vi "Add Modules.vi"(8 "error in (no error)":errorcluster, 10 "Modules in":refnum<k24>[](array[refnum]), 11 "Item Ref in":T1 format="%.0x") -> (0 "error out":errorcluster, 2 "Modules out":refnum<k24>[](array[refnum]), 3 "Item Ref out":T1 format="%.0x")   [LabVIEW 2014, in "SLSC configuration System Explorer.lvlib"]
uses:
  SLSC configuration System Explorer.lvlib
  C:/Files/Custom VeriStand Development/DET-SPI-Tool/XML Deserializer/SLSC Deserializer/SLSC Deserializer/bin/Release/SLSC Deserializer.dll
  XML Deserializer/SLSC Deserializer/SLSC Deserializer/bin/Release/SLSC Deserializer.dll
  <vilib>/NI Veristand/Custom Device API/Custom Device Item Ref.ctl
  Type Defs/Card Position.ctl
  Shared/SPI Utility/Slot #.ctl
  Shared/SLSC configuration Shared.lvlib
  <vilib>/NI Veristand/Custom Device API/Custom Device API.lvlib
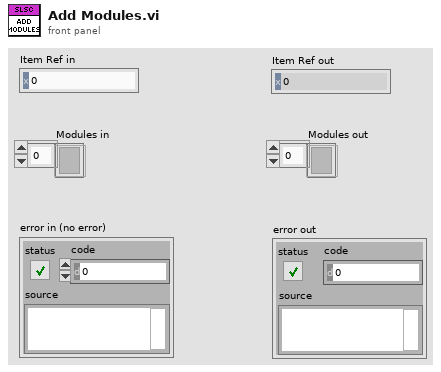
[diagram p1: front panel]
types:
  T1 = typedef "Custom Device API.lvlib/Custom Device Item Ref.ctl" = u64
  T2 = typedef "SLSC configuration Shared.lvlib/Card Position.ctl" = cluster{"Rack #":u8, "Slot #":T3}
  T3 = typedef "SLSC configuration Shared.lvlib/Slot #.ctl" = u8
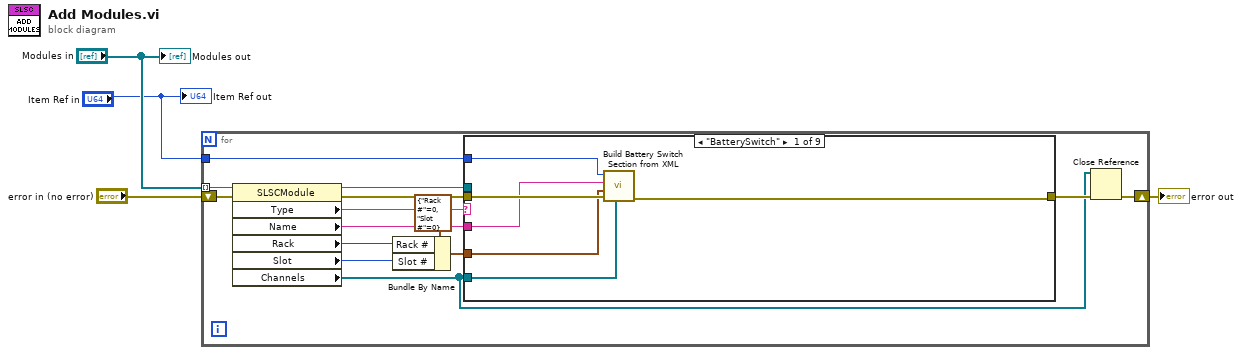
[diagram p0: block diagram]
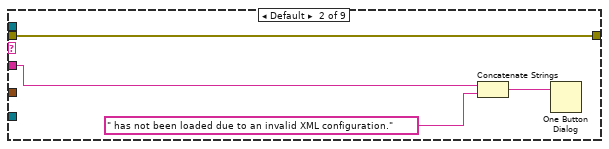
[diagram p2: hidden frame]
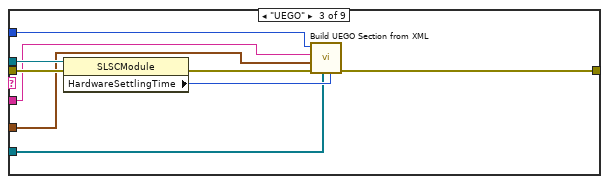
[diagram p3: hidden frame]
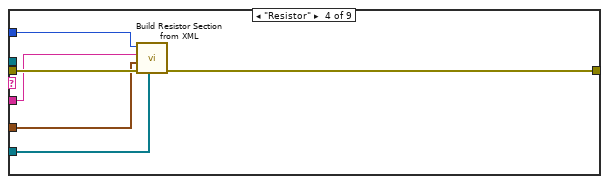
[diagram p4: hidden frame]
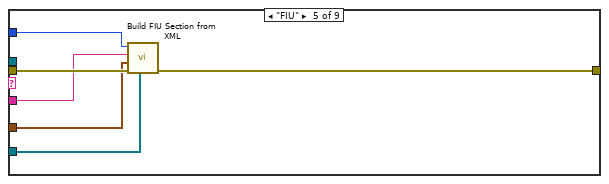
[diagram p5: hidden frame]
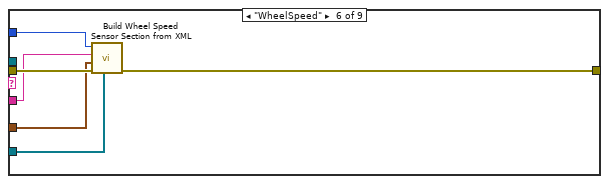
[diagram p6: hidden frame]
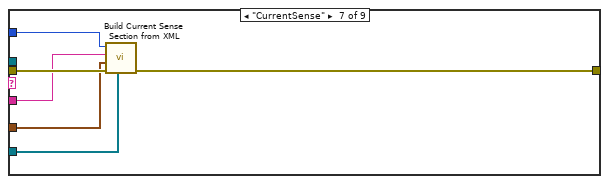
[diagram p7: hidden frame]
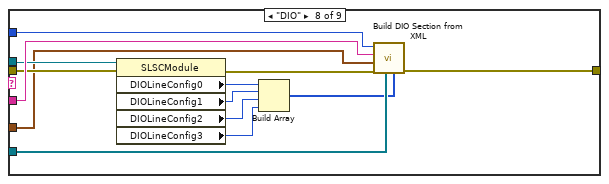
[diagram p8: hidden frame]
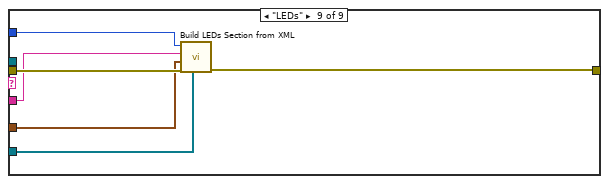
[diagram p9: hidden frame]
diagram:
  n1 = for {
    tunnel: "Modules in" -> [w18] mode=indexing
    shift-right: [w5] -> w2
    shift-left: "error in (no error)" -> [w17]
    tunnel: "Item Ref in" -> [w13]
    n2 = property class="SLSCModule"(reference=w18, error in=w17) -> (reference out=w14:refnum<k24>, error out=w15:errorcluster, "Type"=w16:string, "Name"=w12:string, "Rack"=w10:u8, "Slot"=w9:u8, "Channels"=w6:refnum<k24>[])
    n3 = Bundle By Name(cluster=T2 {"Rack #"=0, "Slot #"=0} ("Card Position in"), "Rack #"=w10, "Slot #"=w9) -> (w8:T2)
    n4 = case shown="\"BatterySwitch\"" w16 {
      tunnel: w15 -> [w24 w25 w37 w43 w49 w55 w61 w71 w80]
      tunnel: w14 -> [_ _ w36 _ _ _ _ w70 _]
      tunnel: w13 -> [w23 _ w34 w42 w48 w54 w59 w73 w79]
      tunnel: w12 -> [w22 w26 w33 w41 w47 w53 w58 w74 w78]
      tunnel: w6 -> [w20 _ w29 w39 w45 w51 w56 w72 w76]
      tunnel: [w19 w25 w30 w38 w44 w50 w60 w63 w75] -> w7
      tunnel: w8 -> [w21 _ w32 w40 w46 w52 w57 w62 w77]
      frame "BatterySwitch" {
        n5 = call "Build Battery Switch Section from XML.vi"("Channels"=w20, "error in (no error)"=w24, "Card Position in"=w21, "Name in"=w22, "Node Ptr in"=w23) -> ("error out"=w19:errorcluster)  [unwired: 6 in]
      }
      frame Default {
        n6 = Concatenate Strings(w26, " has not been loaded due to an invalid XML configuration." ("string")) -> (w27:string)
        n7 = One Button Dialog(message=w27) -> ()  [unwired: 1 in, 1 out]
      }
      frame "UEGO" {
        n8 = property class="SLSCModule"(reference=w36, error in=w37) -> (error out=w35:errorcluster, "HardwareSettlingTime"=w31:u32)  [unwired: 1 out]
        n9 = call "Build UEGO Section from XML.vi"("HW Settling Time"=w31, "Channels"=w29, "error in (no error)"=w35, "Card Position in"=w32, "Name in"=w33, "Node Ptr in"=w34) -> ("error out"=w30:errorcluster)  [unwired: 5 in]
      }
      frame "Resistor" {
        n10 = call "Build Resistor Section from XML.vi"("Channels"=w39, "error in (no error)"=w43, "Card Position"=w40, "Name"=w41, "Node Ptr"=w42) -> ("error out"=w38:errorcluster)  [unwired: 6 in]
      }
      frame "FIU" {
        n11 = call "Build FIU Section from XML.vi"("Channels"=w45, "error in (no error)"=w49, "Card Position in"=w46, "Name in"=w47, "Node Ptr in"=w48) -> ("error out"=w44:errorcluster)  [unwired: 6 in]
      }
      frame "WheelSpeed" {
        n12 = call "Build Wheel Speed Sensor Section from XML.vi"("Channels"=w51, "error in (no error)"=w55, "Card Position in"=w52, "Name in"=w53, "Node Ptr in"=w54) -> ("error out"=w50:errorcluster)  [unwired: 6 in]
      }
      frame "CurrentSense" {
        n13 = call "Build Current Sense Section from XML.vi"("Channels"=w56, "error in (no error)"=w61, "Card Position in"=w57, "Name in"=w58, "Node Ptr in"=w59) -> ("error out"=w60:errorcluster)  [unwired: 6 in]
      }
      frame "DIO" {
        n14 = property class="SLSCModule"(reference=w70, error in=w71) -> (error out=w64:errorcluster, "DIOLineConfig0"=w69:u8, "DIOLineConfig1"=w68:u8, "DIOLineConfig2"=w67:u8, "DIOLineConfig3"=w66:u8)  [unwired: 1 out]
        n15 = Build Array(w69, w68, w67, w66) -> (w65:u8[])
        n16 = call "Build DIO Section from XML.vi"("DIO Line Configs"=w65, "Channels"=w72, "error in (no error)"=w64, "Card Position in"=w62, "Name in"=w74, "Node Ptr in"=w73) -> ("error out"=w63:errorcluster)  [unwired: 5 in]
      }
      frame "LEDs" {
        n17 = call "Build LEDs Section from XML.vi"("Channels"=w76, "error in (no error)"=w80, "Card Position in"=w77, "Name in"=w78, "Node Ptr in"=w79) -> ("error out"=w75:errorcluster)  [unwired: 6 in]
      }
    }
    n18 = Close Reference(reference=w6, error in (no error)=w7) -> (error out=w5:errorcluster)
  }
  "error out" <- w2
  "Modules out" <- "Modules in"
  "Item Ref out" <- "Item Ref in"
